vi "Levelmeter_readout.vi"(7 "VISA-Ressourcenname":refnum<visa-resource-name>) -> (0 "LN Shield Dewar [%]":dbl format="%#_13g", 1 "Coldtrap Dewar [%]":dbl format="%#_13g", 2 "Cold trap [%]":dbl format="%#_13g", 3 "LN Shield [%]":dbl format="%#_13g", 4 "VISA-Ressourcenname 2":refnum<visa-resource-name>, 10 "error out":errorcluster {"code" format="%.0x"})   [LabVIEW 2018]
uses:
  <vilib>/Instr/_visa.llb/VISA Configure Serial Port (Instr).vi
panel:
  out "String":string
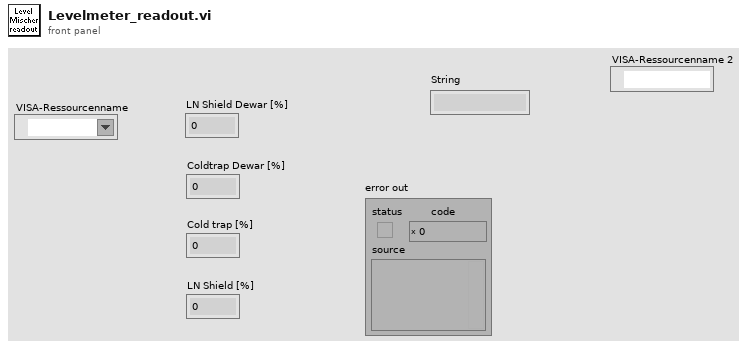
[diagram p1: front panel]
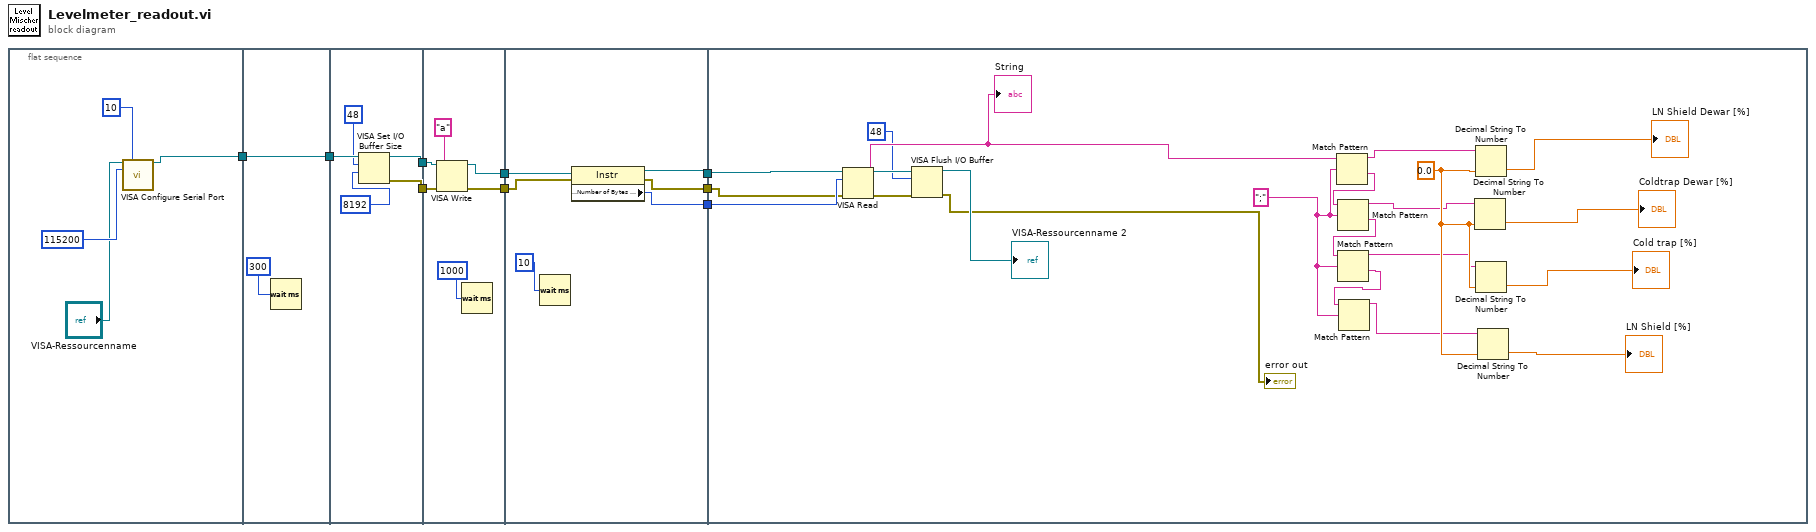
[diagram p0: block diagram]
diagram:
  n1 = flat-sequence {
    tunnel: [w10] -> w2
    tunnel: w2 -> [w15]
    tunnel: [w15] -> w1
    tunnel: [w19] -> w5
    tunnel: [w18] -> w4
    tunnel: w1 -> [w20]
    tunnel: [w23] -> w7
    tunnel: [w22] -> w6
    tunnel: w5 -> [w25]
    tunnel: w4 -> [w24]
    tunnel: [w28] -> w9
    tunnel: w7 -> [w30]
    tunnel: [w29] -> w8
    tunnel: w6 -> [w31]
    tunnel: [w27] -> w3
    tunnel: w9 -> [w38]
    tunnel: w8 -> [w39]
    tunnel: w3 -> [w41]
    frame #0 {
      n2 = call-poly "VISA Configure Serial Port"("VISA resource name"="VISA-Ressourcenname", "timeout (10sec)"=u8 10 ("termination char\n(0xA = '\\n' = LF)"), "baud rate (9600)"=115200) -> ("VISA resource name out"=w10:refnum<visa-resource-name>)  [unwired: 11 in, 1 out]
    }
    frame #1 {
      n3 = Wait (ms)(milliseconds to wait=300) -> ()  [unwired: 1 out]
    }
    frame #2 {
      n4 = VISA Set I/O Buffer Size(VISA resource name=w20, mask (16)=u16 48, size (4096)=u32 8192) -> (VISA resource name out=w18:refnum<visa-resource-name>, error out=w19:errorcluster)  [unwired: 1 in]
    }
    frame #3 {
      n5 = VISA Write(VISA resource name=w24, write buffer="a", error in (no error)=w25) -> (VISA resource name out=w22:refnum<visa-resource-name>, error out=w23:errorcluster)  [unwired: 1 out]
      n6 = Wait (ms)(milliseconds to wait=1000) -> ()  [unwired: 1 out]
    }
    frame #4 {
      n7 = Wait (ms)(milliseconds to wait=10) -> ()  [unwired: 1 out]
      n8 = property class="Instr"(reference=w31, error in=w30) -> (reference out=w29:refnum<visa-resource-name>, error out=w28:errorcluster, "Serial Settings:Number of Bytes at Serial Port"=w27:u32)
    }
    frame #5 {
      w49 = ";"
      w51 = 0.0
      n9 = VISA Read(VISA resource name=w39, byte count=w41, error in (no error)=w38) -> (VISA resource name out=w37:refnum<visa-resource-name>, read buffer=w40:string, error out=w36:errorcluster)  [unwired: 1 out]
      "String" <- w40
      n10 = VISA Flush I/O Buffer(VISA resource name=w37, mask (16)=u16 48, error in (no error)=w36) -> (VISA resource name out=→"VISA-Ressourcenname 2":refnum<visa-resource-name>, error out=→"error out":errorcluster)
      n11 = Match Pattern(string=w40, regular expression=w49) -> (before substring=w45:string, after substring=w48:string)  [unwired: 1 in, 2 out]
      n12 = Match Pattern(string=w48, regular expression=w49) -> (before substring=w44:string, after substring=w47:string)  [unwired: 1 in, 2 out]
      n13 = Match Pattern(string=w47, regular expression=w49) -> (before substring=w43:string, after substring=w46:string)  [unwired: 1 in, 2 out]
      n14 = Match Pattern(string=w46, regular expression=w49) -> (before substring=w50:string)  [unwired: 1 in, 3 out]
      n15 = Decimal String To Number(string=w44, default (0L)=w51) -> (number=→"Coldtrap Dewar [%]":dbl)  [unwired: 1 in, 1 out]
      n16 = Decimal String To Number(string=w45, default (0L)=w51) -> (number=→"LN Shield Dewar [%]":dbl)  [unwired: 1 in, 1 out]
      n17 = Decimal String To Number(string=w43, default (0L)=w51) -> (number=→"Cold trap [%]":dbl)  [unwired: 1 in, 1 out]
      n18 = Decimal String To Number(string=w50, default (0L)=w51) -> (number=→"LN Shield [%]":dbl)  [unwired: 1 in, 1 out]
    }
  }
